vi "Read Parity.vi"(8 "error in (no error)":errorcluster, 11 "Serial Slave in":refnum<class "Serial Slave.lvclass">) -> (0 "error out":errorcluster, 2 "Parity":u16(ring) items=["None", "Odd", "Even", "Mark", "Space"], 3 "Serial Slave out":refnum<class "Serial Slave.lvclass">)   [LabVIEW 2013, in "Modbus Library - Advance.lvlib" / "Serial Slave.lvclass"]
uses:
  Serial Slave.lvclass
  Serial Slave.lvclass/Serial Slave.ctl
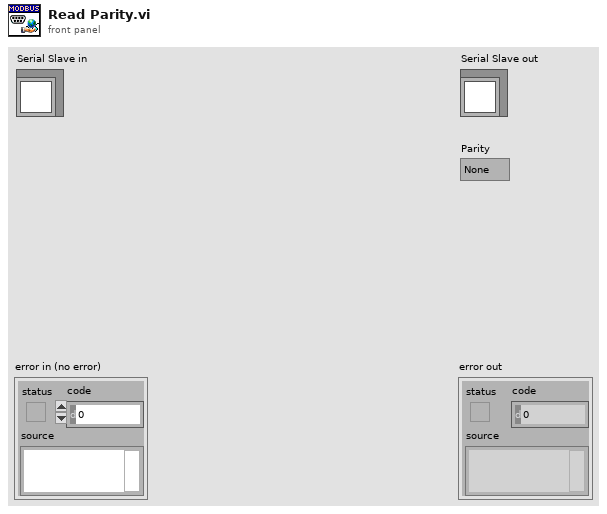
[diagram p1: front panel]
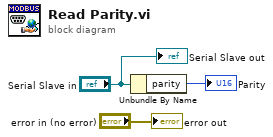
[diagram p0: block diagram]
diagram:
  n1 = Unbundle By Name("Serial Slave in") -> ("parity"=→"Parity":u16)
  "error out" <- "error in (no error)"
  "Serial Slave out" <- "Serial Slave in"
